vi "Init with Shared Options.vi"(5 "Autohide ListBox (F)":bool, 7 "ListBox Refnum (Popup)":refnum<vi>, 8 "error in (no error)":errorcluster, 9 "Height (200)":i16=200, 10 "Shared Options":refnum<class "Shared Options.lvclass">, 11 "Str Refnum":refnum<vi>) -> (0 "error out":errorcluster, 3 "AutoComplete out":refnum<class "AutoComplete.lvclass">)   [LabVIEW 2020, in "AutoComplete.lvlib" / "AutoComplete.lvclass"]
doc: "Initializes an AutoComplete instance similar to <b>Init.vi</b> except that it shares options with other AutoComplete instances using the same Shared Options instance."
uses:
  AutoComplete.lvclass
  Shared Options/Shared Options.lvclass
  AutoComplete.lvclass/AutoComplete.ctl
  AutoComplete.lvlib
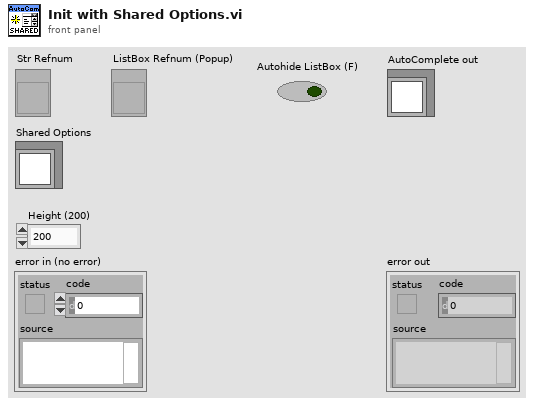
[diagram p1: front panel]
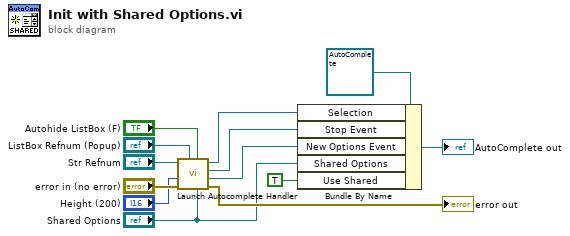
[diagram p0: block diagram]
diagram:
  n1 = call "Launch Autocomplete Handler.vi"("Shared Options (Local)"="Shared Options", "Autohide ListBox (F)"="Autohide ListBox (F)", "ListBox Refnum (Popup)"="ListBox Refnum (Popup)", "error in (no error)"="error in (no error)", "Height (200)"="Height (200)", "Str Refnum"="Str Refnum") -> ("error out"=→"error out":errorcluster, "New Options Event"=w10:refnum<user-event>, "Stop Event"=w11:refnum<user-event>, "Selection"=w12:refnum<user-event>)  [unwired: 2 in]
  n2 = Bundle By Name(cluster=refnum<class "AutoComplete.lvclass"> refnum ("AutoComplete in"), "Selection"=w12, "Stop Event"=w11, "New Options Event"=w10, "Shared Options"="Shared Options", "Use Shared"=TRUE) -> (→"AutoComplete out":refnum<class "AutoComplete.lvclass">)
